vi "toJSON.vi"(8 "error in (no error)":errorcluster, 11 "tBSONRegEx in":refnum<class "tBSONRegEx.lvclass">) -> (0 "error out":errorcluster, 2 "JSON":string, 3 "tBSONRegEx out":refnum<class "tBSONRegEx.lvclass">)   [LabVIEW 2013, in "BSON.lvlib" / "tBSONRegEx.lvclass"]
uses:
  tBSONRegEx.lvclass
  tBSONElement/tBSONElement.lvclass
  getRegularExpression.vi
  getOptionsString.vi
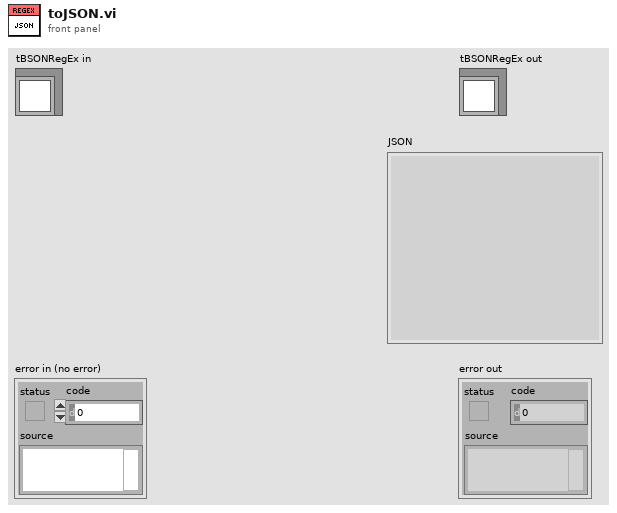
[diagram p1: front panel]
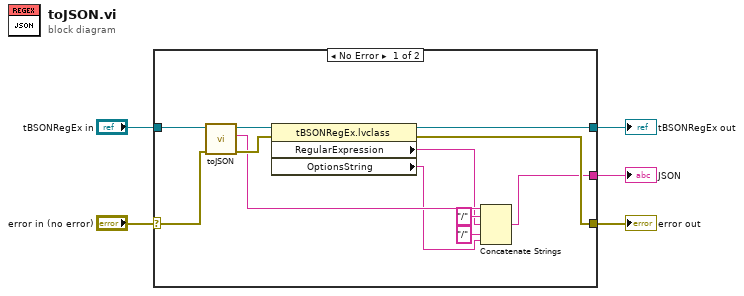
[diagram p0: block diagram]
diagram:
  n1 = case shown="No Error" "error in (no error)" {
    selector: "error in (no error)" -> [w16 w19]
    tunnel: "tBSONRegEx in" -> [w17 w18]
    tunnel: [w12 w19] -> w3
    tunnel: [w14 w18] -> w2
    tunnel: [w6 _] -> w1
    frame No Error {
      n2 = call-parent "toJSON.vi"("error in (no error)"=w16, "tBSONElement in"=w17) -> ("error out"=w13:errorcluster, "JSON"=w11:string, "tBSONElement out"=w15:refnum<class "tBSONRegEx.lvclass">)  [unwired: 7 in]
      n3 = property class="tBSONRegEx.lvclass"(reference=w15, error in=w13) -> (reference out=w14:refnum<class "tBSONRegEx.lvclass">, error out=w12:errorcluster, "RegularExpression"=w9:string, "OptionsString"=w7:string)
      n4 = Concatenate Strings(w11, "/" ("string"), w9, "/" ("string"), w7) -> (w6:string)
    }
    frame Error {
    }
  }
  "error out" <- w3
  "tBSONRegEx out" <- w2
  "JSON" <- w1
